vi "Set Int.vi"(8 "error in (no error)":errorcluster, 10 "Int":i32, 11 "IIntByRef in":refnum<class "IIntByRef (DVR).lvclass">) -> (0 "error out":errorcluster, 3 "IIntByRef out":refnum<class "IIntByRef (DVR).lvclass">)   [LabVIEW 2009, in "IIntByRef (DVR).lvclass"]
uses:
  IIntByRef (DVR).lvclass
  Numeric Test Object.lvclass
  Source/IUnknown Class/IUnknown.lvclass
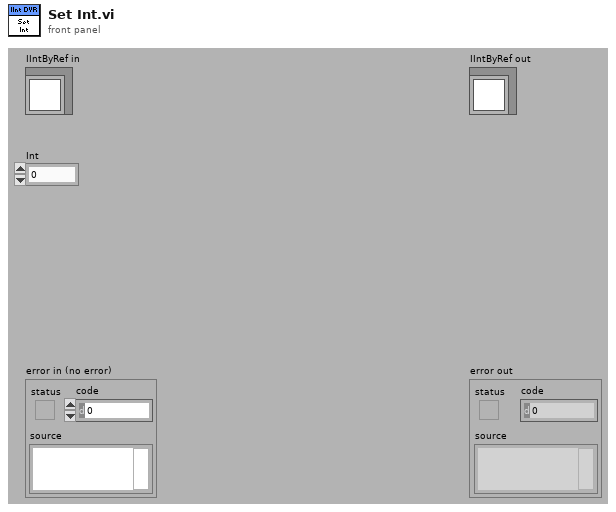
[diagram p1: front panel]
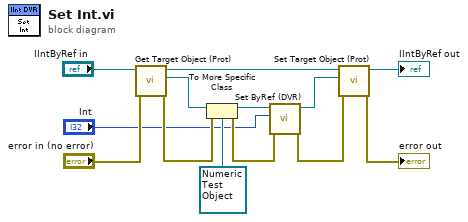
[diagram p0: block diagram]
diagram:
  n1 = call "Get Target Object (Prot).vi"("error in (no error)"="error in (no error)", "IUnknown in"="IIntByRef in") -> ("error out"=w7:errorcluster, "Target Object"=w6:refnum<class "Interfaceable.lvclass">, "IUnknown out"=w12:refnum<class "IIntByRef (DVR).lvclass">)  [unwired: 7 in]
  n2 = To More Specific Class(target class=refnum<class "Numeric Test Object.lvclass"> refnum ("Numeric"), reference=w6, error in=w7) -> (specific class reference=w9:refnum<class "Numeric Test Object.lvclass">, error out=w10:errorcluster)
  n3 = call-dynamic "Set ByRef (DVR).vi"("error in (no error)"=w10, "Int"="Int", "Numeric in"=w9) -> ("error out"=w13:errorcluster, "Numeric out"=w11:refnum<class "Numeric Test Object.lvclass">)  [unwired: 7 in]
  n4 = call "Set Target Object (Prot).vi"("error in (no error)"=w13, "Target Object"=w11, "IUnknown in"=w12) -> ("error out"=→"error out":errorcluster, "IUnknown out"=→"IIntByRef out":refnum<class "IIntByRef (DVR).lvclass">)  [unwired: 7 in]
